vi "Choose Specification.vi"(3 "draft":T1(ring)) -> (1 "draft":string)   [LabVIEW 2019, in "JSON-Schema.lvlib"]
uses:
  JSON-Schema.lvlib
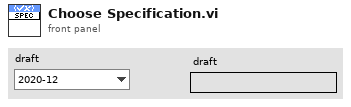
[diagram p1: front panel]
types:
  T1 = enum16{"2020-12", "2019-09", "draft-07", "draft-06", "draft-05"}
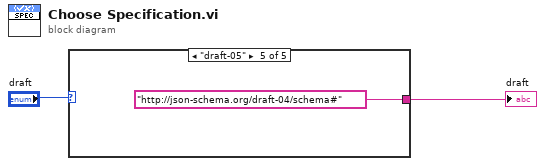
[diagram p0: block diagram]
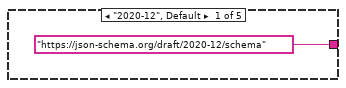
[diagram p2: hidden frame]
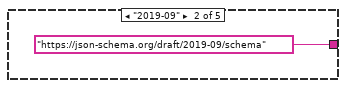
[diagram p3: hidden frame]
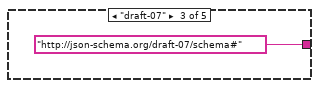
[diagram p4: hidden frame]
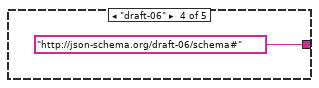
[diagram p5: hidden frame]
diagram:
  n1 = case shown="\"draft-05\"" "draft" {
    tunnel: ["https://json-schema.org/draft/2020-12/schema" ("JSON to Insert") "https://json-schema.org/draft/2019-09/schema" ("JSON to Insert") "http://json-schema.org/draft-07/schema#" ("JSON to Insert") "http://json-schema.org/draft-06/schema#" ("JSON to Insert") "http://json-schema.org/draft-04/schema#" ("JSON to Insert")] -> w2
    frame "2020-12", Default {
    }
    frame "2019-09" {
    }
    frame "draft-07" {
    }
    frame "draft-06" {
    }
    frame "draft-05" {
    }
  }
  "draft" <- w2
